vi "atomNumber.vi"(6 "Image bg":sgl[][](array[numeric]) format="%.2f", 8 "error in (no error)":errorcluster, 9 "Image ref":sgl[][](array[numeric]) format="%.2f", 10 "Image object":sgl[][](array[numeric]) format="%.2f", 11 "BECImageProcessor in":refnum<class "BECImageProcessor.lvclass">) -> (0 "error out":errorcluster, 1 "x width":dbl, 2 "number":dbl, 3 "BECImageProcessor out":refnum<class "BECImageProcessor.lvclass">, 4 "z width":dbl, 5 "Image Out":T1)   [LabVIEW 2009, in "Tools.lvlib" / "Imaging.lvlib" / "BECImageProcessor.lvclass"]
uses:
  BECImageProcessor.lvclass
  <vilib>/vision/Image Controls.llb/IMAQ Image.ctl
  <vilib>/Analysis/NI_AALBase.lvlib
  Compiler.lvlib
panel:
  out "optical density":cluster{i32[], dbl[]}(graph)
  out "reference":cluster{i32[], dbl[]}(graph)
  out "object":cluster{i32[], dbl[]}(graph)
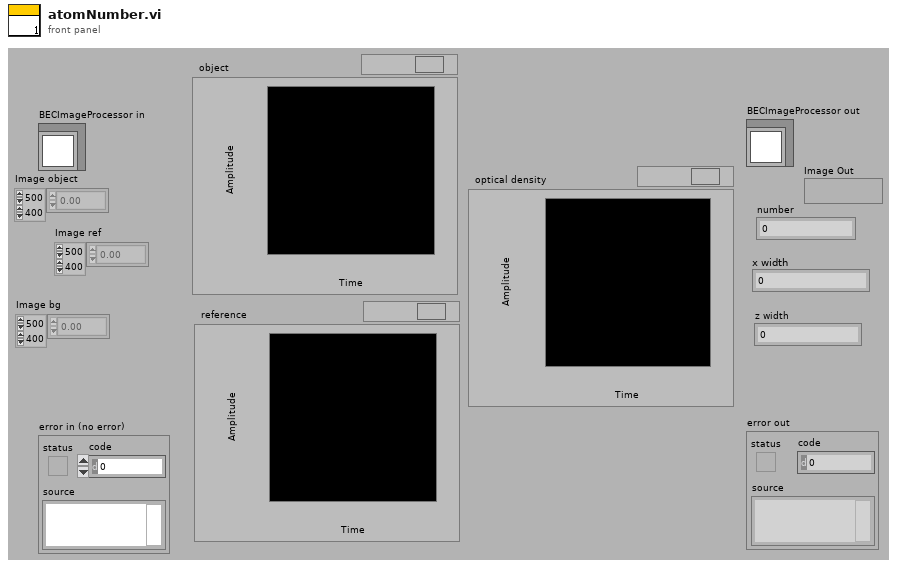
[diagram p1: front panel]
types:
  T1 = typedef "IMAQ Image.ctl" = refnum<image>
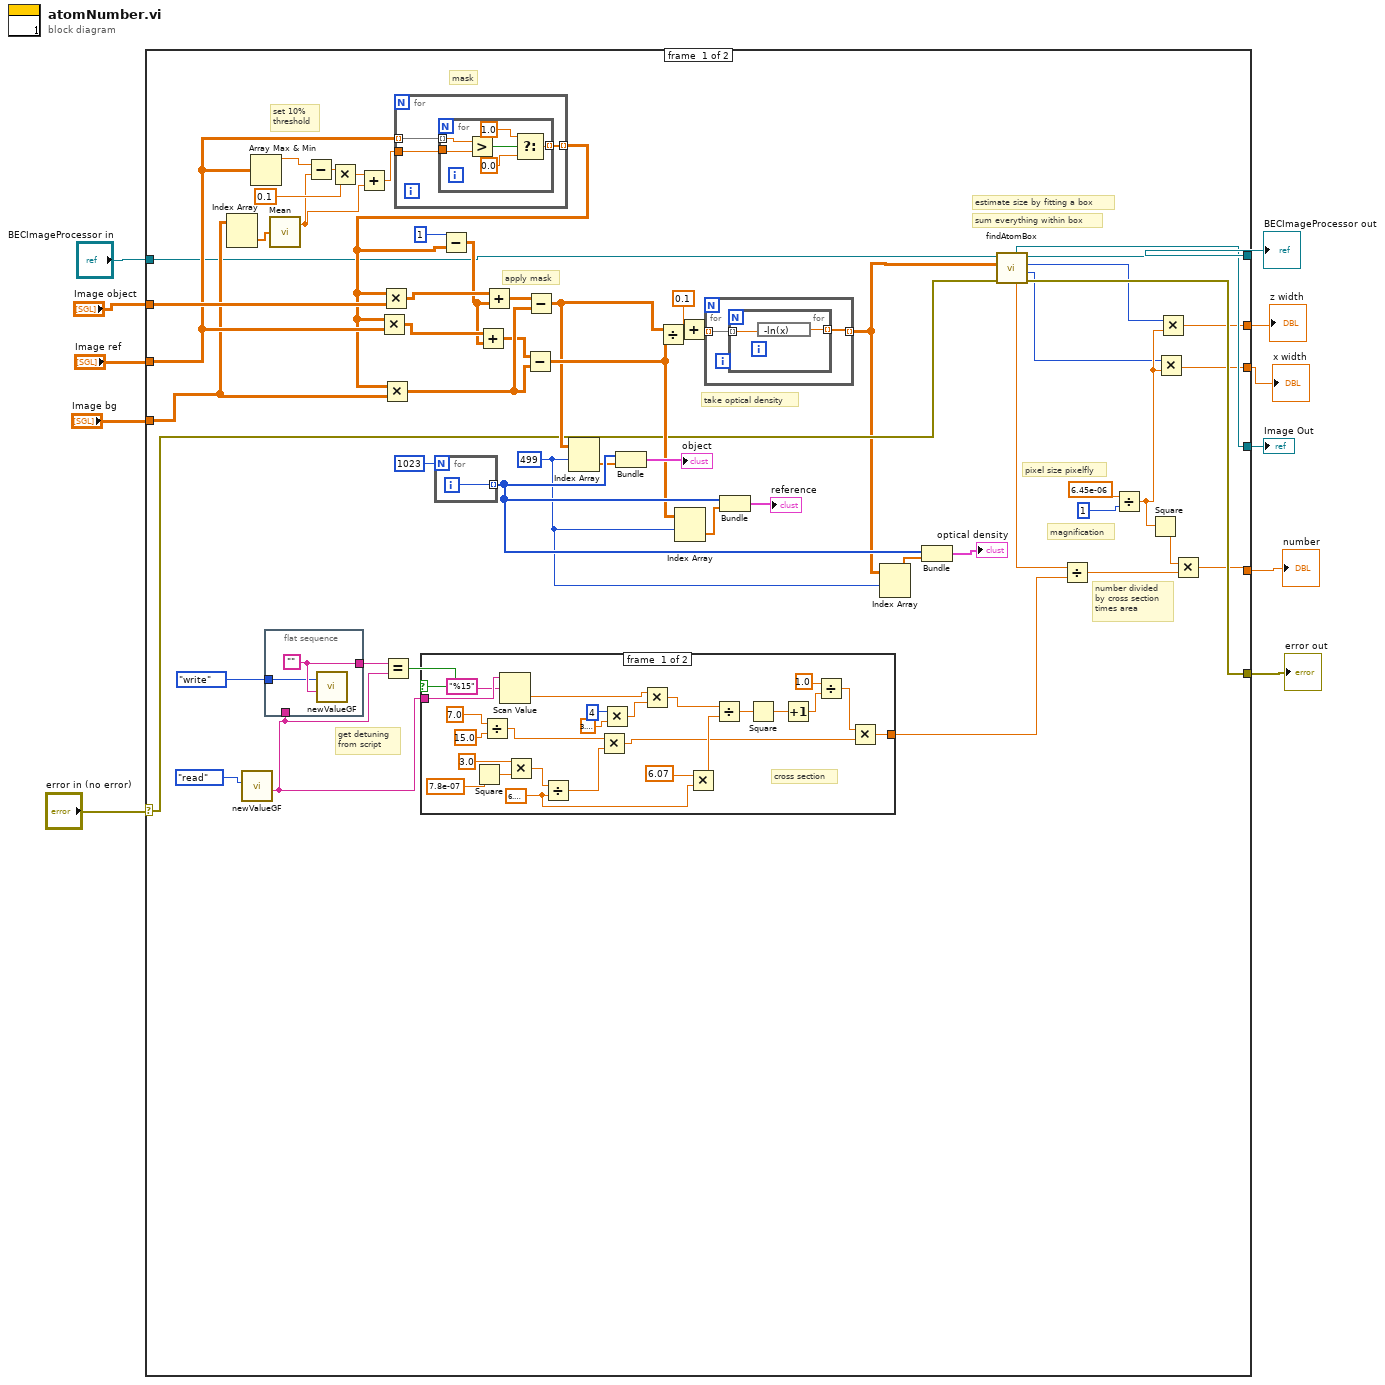
[diagram p0: block diagram]
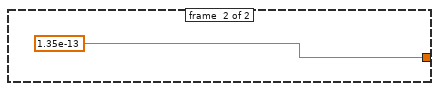
[diagram p2: hidden frame]
diagram:
  n1 = case shown="No Error" "error in (no error)" {
    selector: "error in (no error)" -> [w24 w110]
    tunnel: [w23 w110] -> w10
    tunnel: [w25 w109] -> w8
    tunnel: "BECImageProcessor in" -> [w26 w109]
    tunnel: "Image object" -> [w62 _]
    tunnel: "Image ref" -> [w60 _]
    tunnel: "Image bg" -> [w52 _]
    tunnel: [w16 _] -> w4
    tunnel: [w18 _] -> w3
    tunnel: [w17 _] -> w2
    tunnel: [w19 _] -> w1
    frame #0 {
      w27 = 499
      # "magnification"
      # "pixel size pixelfly"
      # "get detuning\nfrom script"
      # "estimate size by fitting a box"
      # "set 10%\nthreshold"
      # "apply mask"
      # "mask"
      # "number divided\nby cross section\ntimes area"
      # "sum everything within box"
      # "take optical density"
      n2 = Index Array(array=w52) -> (element=w51:sgl[])  [unwired: 2 in]
      n3 = call "newValueGF.vi"("control"=enum16{"read", "write"}."read") -> ("newValue out"=w38:string)  [unwired: 10 in]
      n4 = Array Max & Min(array=w60) -> (max value=w50:sgl)  [unwired: 3 out]
      n5 = flat-sequence {
        tunnel: [w68] -> w40
        tunnel: enum16{"read", "write"}."write" ("control") -> [w67]
        tunnel: w38 -> [_]
        frame #0 {
          w68 = ""
          n6 = call "newValueGF.vi"("newValue"=w68, "control"=w67) -> ()  [unwired: 9 in, 1 out]
        }
      }
      n7 = call <vilib>:"Mean.vi"("X"=w51) -> ("mean"=w34:dbl)  [unwired: 1 out]
      n8 = Subtract(x=w50, y=w34) -> (x-y=w49:dbl)
      n9 = Multiply(x=w49, y=0.1) -> (x*y=w47:dbl)
      n10 = Add(x=w47, y=w34) -> (x+y=w46:dbl)
      n11 = Equal?(x=w40, y=w38) -> (x = y?=w42:bool)
      n12 = for {
        tunnel: w60 -> [w97] mode=indexing
        tunnel: [w96] -> w56 mode=indexing
        tunnel: w46 -> [w95]
        n13 = for {
          tunnel: w97 -> [w103] mode=indexing
          tunnel: w95 -> [w102]
          tunnel: [w98] -> w96 mode=indexing
          n14 = Greater?(x=w103, y=w102) -> (0:w101:bool)
          n15 = Select(t=1.0, s=w101, f=0.0) -> (s? t:f=w98:dbl)
        }
      }
      n16 = Multiply(x=w56, y=w60) -> (x*y=w55:dbl[][])
      n17 = Multiply(x=w56, y=w62) -> (x*y=w58:dbl[][])
      n18 = Multiply(x=w56, y=w52) -> (x*y=w61:dbl[][])
      n19 = case shown="True" w42 {
        tunnel: [w72 1.35e-13] -> w41
        tunnel: w38 -> [w85 _]
        frame #0 {
          w80 = 6.283185307179586
          # "cross section"
          n20 = Square(x=7.8e-07) -> (x^2=w86:dbl)
          n21 = Divide(x=7.0, y=15.0) -> (x/y=w88:dbl)
          n22 = Scan Value(string=w85, format string="%15") -> (value=w83:dbl)  [unwired: 1 in, 1 out]
          n23 = Multiply(x=3.0, y=w86) -> (x*y=w89:dbl)
          n24 = Divide(x=w89, y=w80) -> (x/y=w87:dbl)
          n25 = Multiply(x=w88, y=w87) -> (x*y=w73:dbl)
          n26 = Multiply(x=4, y=3.141592653589793) -> (x*y=w69:dbl)
          n27 = Multiply(x=w83, y=w69) -> (x*y=w82:dbl)
          n28 = Multiply(x=6.07, y=w80) -> (x*y=w79:dbl)
          n29 = Divide(x=w82, y=w79) -> (x/y=w78:dbl)
          n30 = Square(x=w78) -> (x^2=w77:dbl)
          n31 = Increment(x=w77) -> (x+1=w76:dbl)
          n32 = Divide(x=1.0, y=w76) -> (x/y=w74:dbl)
          n33 = Multiply(x=w74, y=w73) -> (x*y=w72:dbl)
        }
        frame #1 {
        }
      }
      n34 = for {
        N: 1023 -> [_]
        tunnel: [w108] -> w35 mode=indexing
        i -> [w108]
      }
      n35 = Subtract(x=1, y=w56) -> (x-y=w54:dbl[][])
      n36 = Add(x=w55, y=w54) -> (x+y=w53:dbl[][])
      n37 = Add(x=w58, y=w54) -> (x+y=w59:dbl[][])
      n38 = Subtract(x=w53, y=w61) -> (x-y=w29:dbl[][])
      n39 = Subtract(x=w59, y=w61) -> (x-y=w28:dbl[][])
      n40 = Index Array(array=w28, index (row)=w27) -> (element=w30:dbl[])  [unwired: 1 in]
      n41 = Bundle(w35, w30) -> (→"object":cluster{i32[], dbl[]})  [unwired: 1 in]
      n42 = Divide(x=w28, y=w29) -> (x/y=w15:dbl[][])
      n43 = Index Array(array=w29, index (row)=w27) -> (element=w33:dbl[])  [unwired: 1 in]
      n44 = Add(x=0.1, y=w15) -> (x+y=w13:dbl[][])
      n45 = for {
        tunnel: w13 -> [w105] mode=indexing
        tunnel: [w104] -> w14 mode=indexing
        n46 = for {
          tunnel: w105 -> [w107] mode=indexing
          tunnel: [w106] -> w104 mode=indexing
          n47 = expression code="-ln(x)"(w107) -> (w106:dbl)
        }
      }
      n48 = Bundle(w35, w33) -> (→"reference":cluster{i32[], dbl[]})  [unwired: 1 in]
      n49 = Index Array(array=w14, index (row)=w27) -> (element=w32:dbl[])  [unwired: 1 in]
      n50 = Bundle(w35, w32) -> (→"optical density":cluster{i32[], dbl[]})  [unwired: 1 in]
      n51 = call "findAtomBox.vi"("error in (no error)"=w24, "imageArray"=w14, "BECImageProcessor in"=w26) -> ("error out"=w23:errorcluster, "y Dimension"=w22:i32, "x Dimension"=w21:i32, "BECImageProcessor out"=w25:refnum<class "BECImageProcessor.lvclass">, "integralNumeric"=w20:dbl, "Image Out"=w19:T1)  [unwired: 3 in]
      n52 = Divide(x=w20, y=w41) -> (x/y=w64:dbl)
      n53 = Divide(x=6.45e-06, y=1) -> (x/y=w44:dbl)
      n54 = Square(x=w44) -> (x^2=w63:dbl)
      n55 = Multiply(x=w22, y=w44) -> (x*y=w17:dbl)
      n56 = Multiply(x=w21, y=w44) -> (x*y=w18:dbl)
      n57 = Multiply(x=w63, y=w64) -> (x*y=w16:dbl)
    }
    frame #1 {
    }
  }
  "error out" <- w10
  "BECImageProcessor out" <- w8
  "x width" <- w2
  "number" <- w4
  "z width" <- w3
  "Image Out" <- w1
